vi "Get angle.vi"(0 "ADI IMU DevRef Out":T1, 1 "Robot":enum16{"Linda/Sophie", "Mule"}(ring)) -> (2 "Out":dbl, 3 "Turn to Home":dbl, 4 "Wraped Out":dbl)   [LabVIEW 2018]
doc: "Get's gyro readings both absolute as well as wrapped"
uses:
  ADIS16448 IMU/ADI_IMU_ADIS16448_IMUDevRef.ctl
  <vilib>/Rock Robotics/SystemInterfaces/spilib/spi_bus.ctl
  Framework/Robot Global Data.vi
  ADIS16448 IMU/ADIS16448_IMU.lvlib
panel:
  out "Angles":cluster{dbl}(graph)
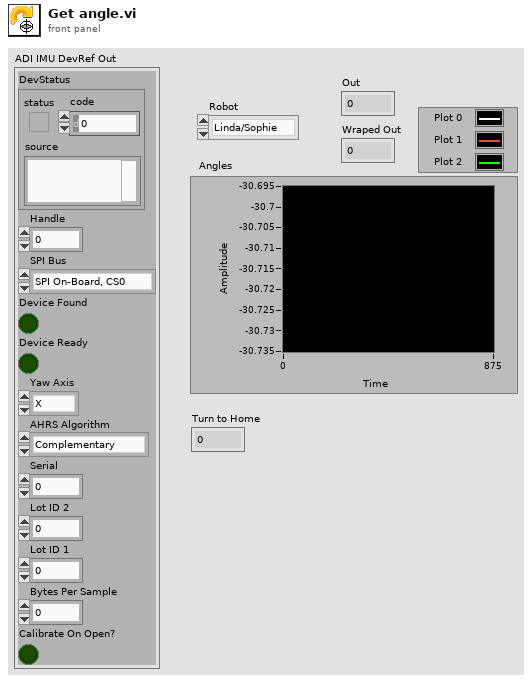
[diagram p1: front panel]
types:
  T1 = typedef "ADIS16448_IMU.lvlib/ADI_IMU_ADIS16448_IMUDevRef.ctl" = cluster{"DevStatus":errorcluster, "Handle":i32, "SPI Bus":T2, "Device Found":bool, "Device Ready":bool, "Yaw Axis":enum16{"X", "Y", "Z"}, "AHRS Algorithm":enum16{"Complementary", "Madgwick"}, "Serial":u16, "Lot ID 2":u16, "Lot ID 1":u16, "Bytes Per Sample":u16, "Calibrate On Open?":bool}
  T2 = typedef "spi_bus.ctl" = enum16{"SPI On-Board, CS0", "SPI On-Board, CS1", "SPI On-Board, CS2", "SPI On-Board, CS3", "SPI MXP", "Invalid"}
  T3 = cluster{"X Angle":dbl, "Y Angle":dbl, "Z Angle":dbl}
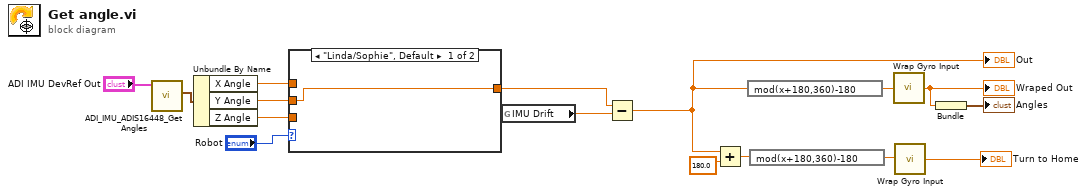
[diagram p0: block diagram]
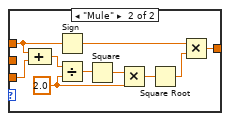
[diagram p2: hidden frame]
diagram:
  n1 = call "ADI_IMU_ADIS16448_Get Angles.vi"("ADI IMU DevRef"="ADI IMU DevRef Out") -> ("IMU Angles Out"=w13:T3)  [unwired: 7 in, 3 out]
  n2 = Unbundle By Name(w13) -> ("X Angle"=w14:dbl, "Y Angle"=w10:dbl, "Z Angle"=w11:dbl)
  n3 = case shown="\"Linda/Sophie\", Default" "Robot" {
    tunnel: [w17 w27] -> w3
    tunnel: w14 -> [_ w23]
    tunnel: w11 -> [_ w18]
    tunnel: w10 -> [w17 _]
    frame "Linda/Sophie", Default {
    }
    frame "Mule" {
      w26 = 2.0 ("y")
      n4 = Compound Arithmetic op=ADD(w23, w18) -> (w24:dbl)
      n5 = Sign(1:w23) -> (0:w21:dbl)
      n6 = Divide(x=w24, y=w26) -> (x/y=w25:dbl)
      n7 = Square(x=w25) -> (x^2=w19:dbl)
      n8 = Multiply(x=w19, y=w26) -> (x*y=w20:dbl)
      n9 = Square Root(x=w20) -> (sqrt(x)=w22:dbl)
      n10 = Multiply(x=w21, y=w22) -> (x*y=w27:dbl)
    }
  }
  n11 = global read "Robot Global Data.vi" "IMU Drift"() -> (w2:dbl)
  n12 = Subtract(x=w3, y=w2) -> (x-y=w1:dbl)
  "Out" <- w1
  n13 = Add(x=w1, y=180.0) -> (x+y=w6:dbl)
  n14 = expression code="mod(x+180,360)-180"(w1) -> (w8:dbl)
  n15 = expression code="mod(x+180,360)-180"(w6) -> (w7:dbl)
  n16 = call "Wrap Gyro Input.vi"("In"=w8) -> ("Out"=w16:dbl)
  "Wraped Out" <- w16
  n17 = call "Wrap Gyro Input.vi"("In"=w7) -> ("Out"=→"Turn to Home":dbl)
  n18 = Bundle("Out"=w16) -> (→"Angles":cluster{"Out":dbl})  [unwired: 1 in]
